vi "Remove Dependent Node ID.vi"(11 "Tree In":T1[](array[typedef]) {"Properties"."Type" items=["K_STRING", "K_BOOL", "K_I32", "K_U32", "K_DOUBLE", "K_U64", "K_VARIANT", "K_DEPENDENTFILE", "K_DEPENDENTNODE", "K_DATASOURCENODE", "K_U16", "K_DBLARR", "K_U32ARR", "K_I32ARR", "K_STRINGARR", "K_DICTIONARY", "K_DICTIONARYARR"]}) -> (3 "Tree Out":T1[](array[typedef]) {"Properties"."Type" items=["K_STRING", "K_BOOL", "K_I32", "K_U32", "K_DOUBLE", "K_U64", "K_VARIANT", "K_DEPENDENTFILE", "K_DEPENDENTNODE", "K_DATASOURCENODE", "K_U16", "K_DBLARR", "K_U32ARR", "K_I32ARR", "K_STRINGARR", "K_DICTIONARY", "K_DICTIONARYARR"]})   [LabVIEW 2020, in "Routing and Faulting Export Unit Tests.lvclass"]
uses:
  Routing and Faulting Export Unit Tests.lvclass
  <vilib>/NI/NI VeriStand Advanced SysDef API/_Types/TreeItem.ctl
  <vilib>/NI/NI VeriStand Advanced SysDef API/_Types/TreeItem.Info.ctl
  <vilib>/NI VeriStand/Custom Device API/Custom Device Channel.ctl
  <vilib>/NI VeriStand/Custom Device API/Custom Device Channel Type.ctl
  <vilib>/NI VeriStand/Custom Device API/Custom Device Waveform.ctl
  <vilib>/NI VeriStand/Custom Device API/Custom Device Waveform DataType.ctl
  <vilib>/NI/NI VeriStand Advanced SysDef API/_Types/TreeItem.Property.ctl
  <vilib>/NI/NI VeriStand Advanced SysDef API/SysDef API/Advanced System Definition.lvlib
  <vilib>/NI VeriStand/Custom Device API/Custom Device API.lvlib
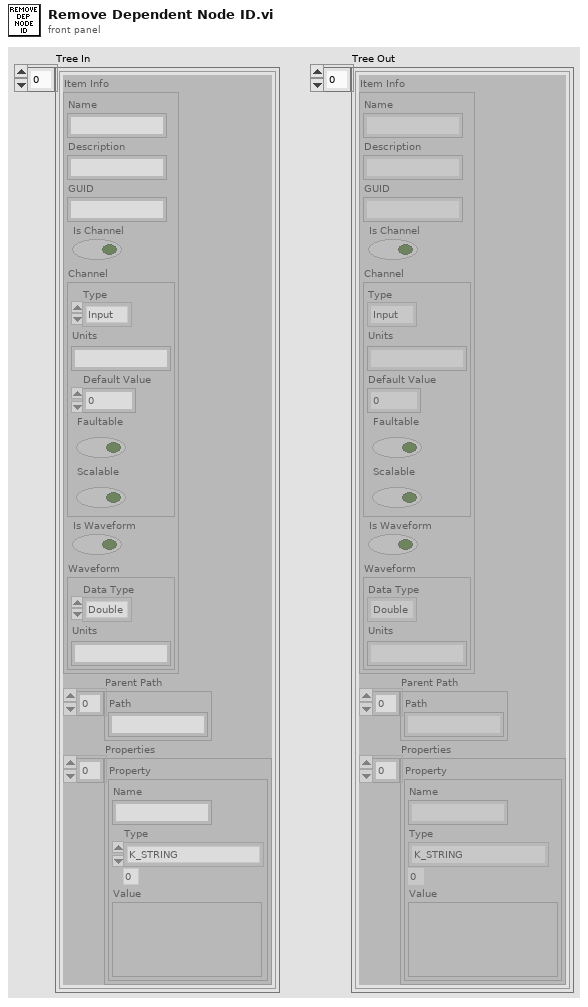
[diagram p1: front panel]
types:
  T1 = typedef "Advanced System Definition.lvlib/TreeItem.ctl" = cluster{"Item Info":T2, "Parent Path":string[], "Properties":T7[]}
  T2 = typedef "Advanced System Definition.lvlib/TreeItem.Info.ctl" = cluster{"Name":string, "Description":string, "GUID":string, "Is Channel":bool, "Channel":T3, "Is Waveform":bool, "Waveform":T5}
  T3 = typedef "Custom Device API.lvlib/Custom Device Channel.ctl" = cluster{"Type":T4, "Units":string, "Default Value":dbl, "Faultable":bool, "Scalable":bool}
  T4 = typedef "Custom Device API.lvlib/Custom Device Channel Type.ctl" = enum16{"Input", "Output"}
  T5 = typedef "Custom Device API.lvlib/Custom Device Waveform.ctl" = cluster{"Data Type":T6, "Units":string}
  T6 = typedef "Custom Device API.lvlib/Custom Device Waveform DataType.ctl" = enum16{"Double", "Complex Double"}
  T7 = typedef "Advanced System Definition.lvlib/TreeItem.Property.ctl" = cluster{"Name":string, "Type":i32, "Value":variant}
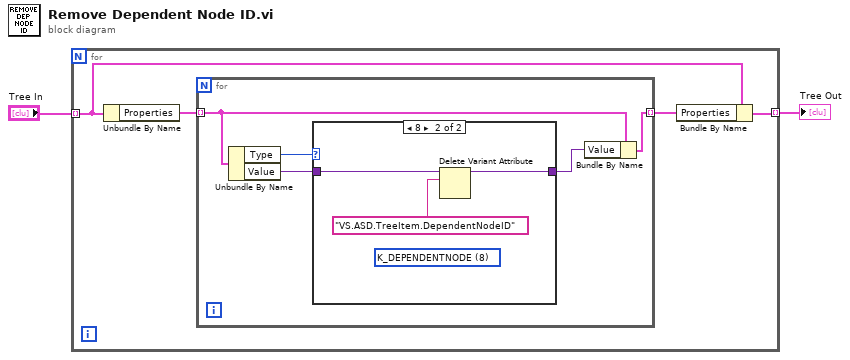
[diagram p0: block diagram]
diagram:
  n1 = for {
    tunnel: "Tree In" -> [w5] mode=indexing
    tunnel: [w3] -> w2 mode=indexing
    n2 = Unbundle By Name(w5) -> ("Properties"=w6:T7[])
    n3 = for {
      tunnel: w6 -> [w9] mode=indexing
      tunnel: [w7] -> w4 mode=indexing
      n4 = Unbundle By Name(w9) -> ("Type"=w10:i32, "Value"=w11:variant)
      n5 = case shown="8" w10 {
        tunnel: w11 -> [w12 w14]
        tunnel: [w12 w13] -> w8
        frame 0, Default {
        }
        frame 8 {
          (unwired) 8 items=["K_STRING", "K_BOOL", "K_I32", "K_U32", "K_DOUBLE", "K_U64", "K_VARIANT", "K_DEPENDENTFILE", "K_DEPENDENTNODE", "K_DATASOURCENODE", "K_U16", "K_DBLARR", "K_U32ARR", "K_I32ARR", "K_STRINGARR", "K_DICTIONARY", "K_DICTIONARYARR"] ("Type")
          n6 = Delete Variant Attribute(6:"VS.ASD.TreeItem.DependentNodeID" ("name"), 7:w14) -> (3:w13:variant)  [unwired: 1 in, 2 out]
        }
      }
      n7 = Bundle By Name(cluster=w9, "Value"=w8) -> (w7:T7)
    }
    n8 = Bundle By Name(cluster=w5, "Properties"=w4) -> (w3:T1)
  }
  "Tree Out" <- w2
